vi "mov_relat.vi"(0 "Board ID":T3=1 min=1 max=32 step=1, 2 "Target Position (0)":i32, 5 "Axis or Vector Space":T2=1 items=["Axis 1"=1, "Axis 2"=2, "Axis 3"=3, "Axis 4"=4, "Axis 5"=5, "Axis 6"=6, "Axis 7"=7, "Axis 8"=8, "Vector Space 1"=17, "Vector Space 2"=18, "Vector Space 3"=19, "Vector Space 4"=20], 7 "Velocity (10000)":i32=10000 min=-20000000 max=20000000, 9 "Acceleration (100000)":u32=100000, 11 "error in (no error)":errorcluster) -> (4 "Bd ID Out":T1, 15 "error out":errorcluster)   [LabVIEW 2016]
uses:
  <vilib>/Motion/FlexMotion/CustomControls/CustomControls.llb/AxisOrVectorSpace To Configure.flx
  <vilib>/Motion/FlexMotion/FunctionsVIs/Trajectory.llb/Load Acceleration/Deceleration.flx
  <vilib>/Motion/FlexMotion/FunctionsVIs/StartStopMotion.llb/Start Motion (8 axes).flx
  <vilib>/Motion/FlexMotion/FunctionsVIs/Trajectory.llb/Check Move Complete Status (8 axes).flx
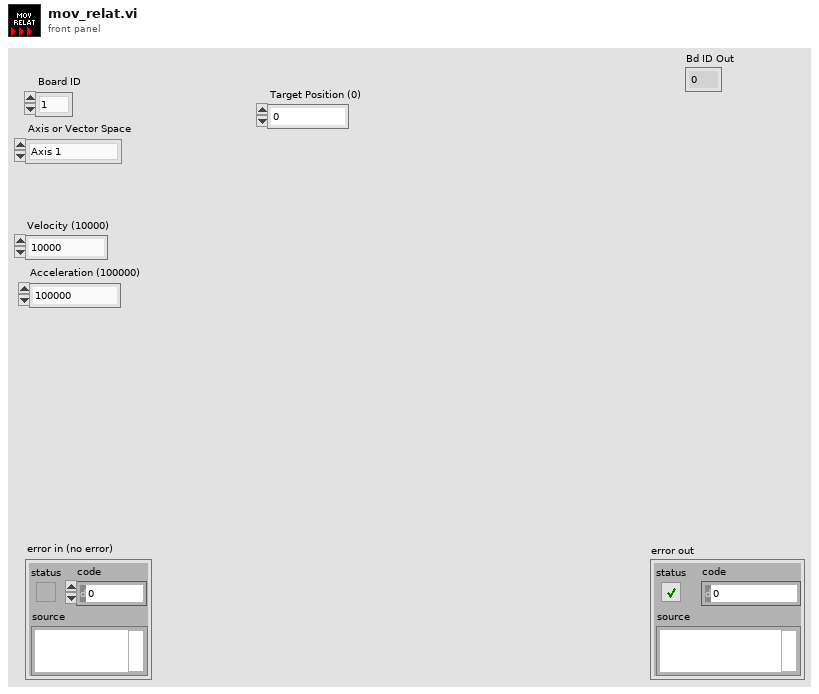
[diagram p1: front panel]
types:
  T1 = typedef "Bd Id Out" = u8
  T2 = typedef "AxisOrVectorSpace To Configure.flx" = u16
  T3 = typedef "Board Id" = u8
  T4 = enum16{"Absolute Position", "Relative Position", "Velocity", "Relative to Cap Pos", "Modulus Position", "Absolute Contouring", "Relative Contouring"}
  T5 = typedef "Resource Out (Enum).flx" = u16
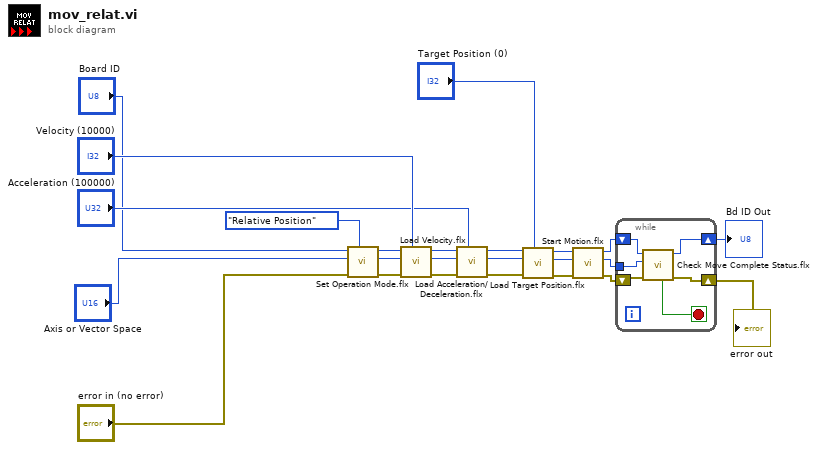
[diagram p0: block diagram]
diagram:
  n1 = call <vilib>:"Set Operation Mode.flx"("Position Mode (Absolute)"=T4."Relative Position", "error in (no error)"="error in (no error)", "Axis or Vector Space"="Axis or Vector Space", "Board ID"="Board ID") -> ("error out"=w22:errorcluster, "Resource Output"=w23:T5, "Bd ID Out"=w24:T1)  [unwired: 2 in]
  n2 = call <vilib>:"Load Velocity.flx"("Velocity (10000)"="Velocity (10000)", "error in (no error)"=w22, "Axis or Vector Space"=w23, "Board ID"=w24) -> ("error out"=w17:errorcluster, "Resource Output"=w18:T5, "Bd ID Out"=w19:T1)  [unwired: 3 in]
  n3 = call "Load Acceleration/Deceleration.flx"("Acceleration (100000)"="Acceleration (100000)", "error in (no error)"=w17, "Axis or Vector Space"=w18, "Board ID"=w19) -> ("error out"=w13:errorcluster, "Resource Output"=w14:T5, "Bd ID Out"=w15:T1)  [unwired: 3 in]
  n4 = call <vilib>:"Load Target Position.flx"("Target Position (0)"="Target Position (0)", "error in (no error)"=w13, "Axis"=w14, "Board ID"=w15) -> ("error out"=w10:errorcluster, "Resource Output"=w11:T5, "Bd ID Out"=w12:T1)  [unwired: 3 in]
  n5 = call-poly <vilib>:"Start Motion.flx"("error in (no error)"=w10, "Axis or Vector Space"=w11, "Board ID"=w12) -> ("error out"=w7:errorcluster, "Resource Output"=w8:T5, "Bd ID Out"=w9:T1)  [unwired: 3 in]
  n6 = while {
    tunnel: w8 -> [w29]
    shift-right: [w27] -> w2
    shift-left: w9 -> [w30]
    shift-right: [w26] -> w1
    shift-left: w7 -> [w28]
    stop <- w25 stop-if-true
    n7 = call-poly <vilib>:"Check Move Complete Status.flx"("error in (no error)"=w28, "Axis or Vector Space"=w29, "Board ID"=w30) -> ("error out"=w26:errorcluster, "Bd ID Out"=w27:T1, "Move Complete"=w25:bool)  [unwired: 3 in, 1 out]
  }
  "Bd ID Out" <- w2
  "error out" <- w1
